vi "PowerMeter-Sample.vi"() -> ()   [LabVIEW 2014]
panel:
  out "Waveform Chart":u32(graph)=11
  out "delay (ms)":u32=11
  out "Active":bool
  in  "stop":bool
  out "Power Value":dbl=-5.48188109e-05 caption="Optical Power [W]" format="%#_4p"
  # "TLPM"
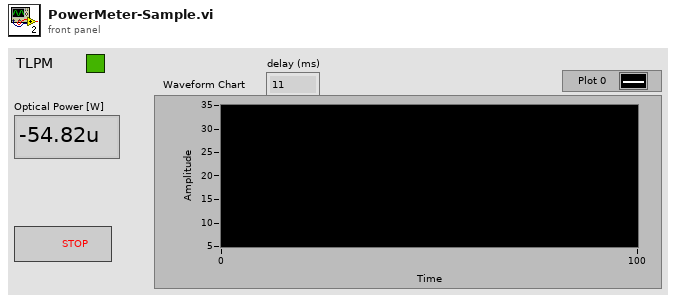
[diagram p1: front panel]
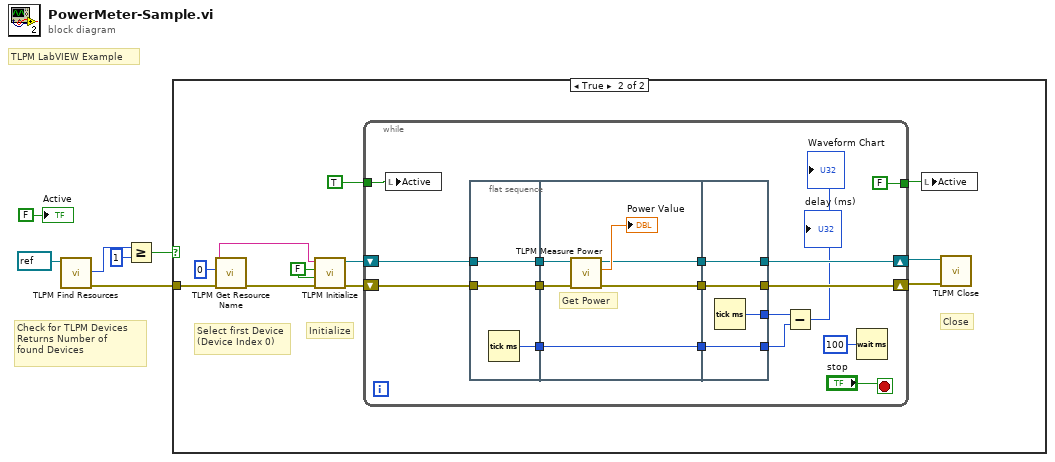
[diagram p0: block diagram]
diagram:
  # "TLPM LabVIEW Example"
  # "Check for TLPM Devices\nReturns Number of\nfound Devices"
  n1 = call "TLPM Find Resources.vi"("instrument handle"=refnum<visa-resource-name> refnum) -> ("error out"=w5:errorcluster, "Resource Count"=w3:u32)  [unwired: 8 in, 1 out]
  n2 = Greater Or Equal?(x=w3, y=u32 1) -> (x >= y?=w4:bool)
  n3 = case shown="True" w4 {
    tunnel: w5 -> [_ w13]
    frame False {
    }
    frame True {
      w11 = FALSE ("ID Query (Do Query)")
      # "Close"
      # "Initialize"
      # "Select first Device\n(Device Index 0)"
      n4 = call "TLPM Get Resource Name.vi"("error in (no error)"=w13, "Index (0)"=u32 0 ("Device Index")) -> ("error out"=w16:errorcluster, "Resource Name"=w14:string)  [unwired: 7 in, 1 out]
      n5 = call "TLPM Initialize.vi"("error in (no error)"=w16, "Reset Device (Reset Device)"=w11, "ID Query (Do Query)"=w11, "resource name"=w14) -> ("error out"=w9:errorcluster, "instrument handle out"=w10:refnum<visa-resource-name>)  [unwired: 6 in]
      n6 = while {
        shift-right: [w28] -> w17
        shift-left: w10 -> [w34]
        shift-right: [w27] -> w15
        shift-left: w9 -> [w33]
        tunnel: [FALSE ("Active")] -> w8
        tunnel: TRUE ("Active") -> [w29]
        stop <- "stop" stop-if-true
        n7 = local write "Active"(w29) -> ()
        n8 = flat-sequence {
          tunnel: w33 -> [w36]
          tunnel: w34 -> [w37]
          tunnel: [w37] -> w24
          tunnel: [w36] -> w23
          tunnel: [w35] -> w21
          tunnel: [w40] -> w26
          tunnel: [w39] -> w25
          tunnel: w24 -> [w42]
          tunnel: w23 -> [w41]
          tunnel: w21 -> [w38]
          tunnel: [w38] -> w20
          tunnel: [w46] -> w27
          tunnel: [w47] -> w28
          tunnel: w26 -> [w47]
          tunnel: w25 -> [w46]
          tunnel: [w45] -> w22
          tunnel: w20 -> [w44]
          tunnel: [w44] -> w19
          frame #0 {
            n9 = Tick Count (ms)() -> (millisecond timer value=w35:u32)
          }
          frame #1 {
            # "Get Power"
            n10 = call "TLPM Measure Power.vi"("error in (no error)"=w41, "instrument handle"=w42) -> ("error out"=w39:errorcluster, "Power"=→"Power Value":dbl, "instrument handle out"=w40:refnum<visa-resource-name>)  [unwired: 7 in]
          }
          frame #2 {
            n11 = Tick Count (ms)() -> (millisecond timer value=w45:u32)
          }
        }
        n12 = Subtract(x=w22, y=w19) -> (x-y=→"delay (ms)" →"Waveform Chart":u32)
        n13 = Wait (ms)(milliseconds to wait=u32 100) -> ()  [unwired: 1 out]
      }
      n14 = local write "Active"(w8) -> ()
      n15 = call "TLPM Close.vi"("error in (no error)"=w15, "instrument handle"=w17) -> ()  [unwired: 9 in, 1 out]
    }
  }
  "Active" <- FALSE ("Active")
